vi "Configure Measurement.vi"(8 "error in (no error)":errorcluster, 11 "Cap Bank Interface in":refnum<class "Cap Bank Interface.lvclass">) -> (0 "error out":errorcluster, 3 "Cap Bank Interface out":refnum<class "Cap Bank Interface.lvclass">)   [LabVIEW 2015, in "Cap Bank Interface.lvclass"]
uses:
  Cap Bank Interface.lvclass
  Cap Bank Interface.lvclass/Cap Bank Interface.ctl
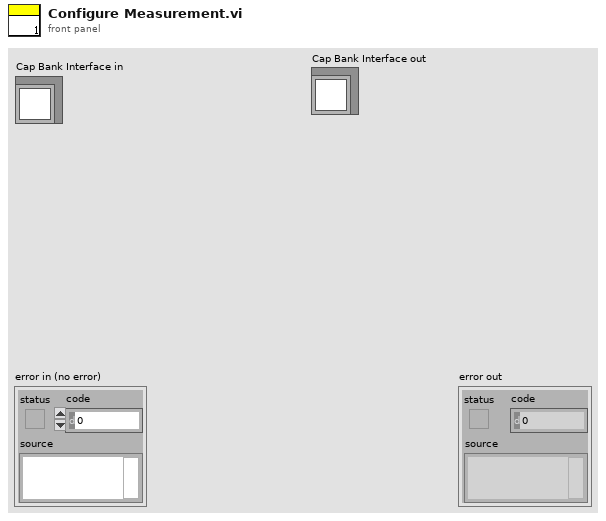
[diagram p1: front panel]
types:
  T1 = typedef "OPC Adresses.ctl" = cluster{"Data Received  URL":string, "Data Ready URL":string, "Message URL":string}
  T2 = typedef "OPC connections.ctl" = cluster{"Data received":refnum<k13>, "Data Ready":refnum<k13>, "Message":refnum<k13>}
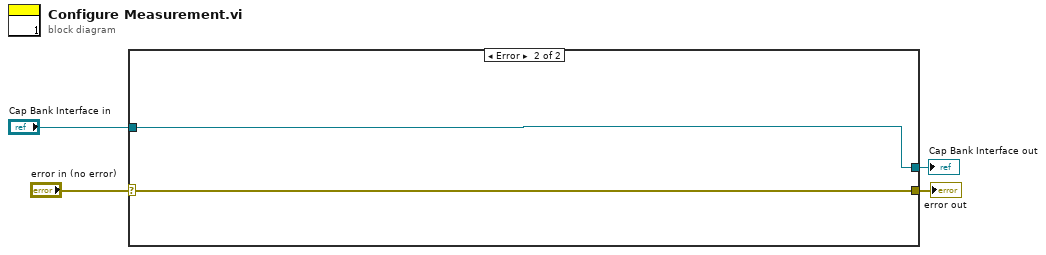
[diagram p0: block diagram]
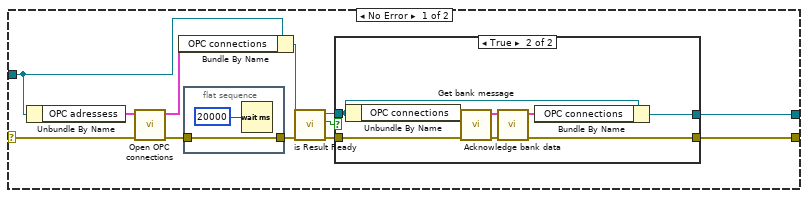
[diagram p2: hidden frame]
diagram:
  n1 = case shown="Error" "error in (no error)" {
    selector: "error in (no error)" -> [w14 w30]
    tunnel: [w6 w30] -> w3
    tunnel: "Cap Bank Interface in" -> [w16 w29]
    tunnel: [w5 w29] -> w1
    frame No Error {
      n2 = Unbundle By Name(w16) -> ("OPC adressess"=w15:T1)
      n3 = call "Open OPC connections.vi"("error in (no error)"=w14, "OPC adressess"=w15) -> ("error IO"=w12:errorcluster, "OPC connections"=w13:T2)  [unwired: 8 in]
      n4 = Bundle By Name(cluster=w16, "OPC connections"=w13) -> (w10:refnum<class "Cap Bank Interface.lvclass">)
      n5 = flat-sequence {
        tunnel: w12 -> [w27]
        tunnel: [w27] -> w11
        frame #0 {
          n6 = Wait (ms)(milliseconds to wait=u32 20000) -> ()  [unwired: 1 out]
        }
      }
      n7 = call-dynamic "is Result Ready.vi"("error in (no error)"=w11, "Cap Bank Interface in"=w10) -> ("error out"=w9:errorcluster, "Result Available"=w8:bool, "Cap Bank Interface out"=w7:refnum<class "Cap Bank Interface.lvclass">)  [unwired: 7 in]
      n8 = case shown="True" w8 {
        tunnel: w9 -> [w17 w22]
        tunnel: w7 -> [w18 w20]
        tunnel: [w17 w21] -> w6
        tunnel: [w18 w19] -> w5
        frame False {
        }
        frame True {
          n9 = Unbundle By Name(w20) -> ("OPC connections"=w26:T2)
          n10 = call "Get bank message.vi"("error IO"=w22, "OPC connections"=w26) -> ("error out"=w23:errorcluster, "OPC connections out"=w25:T2)  [unwired: 4 in, 4 out]
          n11 = call "Acknowledge bank data.vi"("error in"=w23, "OPC connections"=w25) -> ("error out"=w21:errorcluster, "OPC connections out"=w24:T2)  [unwired: 7 in, 1 out]
          n12 = Bundle By Name(cluster=w20, "OPC connections"=w24) -> (w19:refnum<class "Cap Bank Interface.lvclass">)
        }
      }
    }
    frame Error {
    }
  }
  "error out" <- w3
  "Cap Bank Interface out" <- w1
